vi "Load Config_Palette Data.vi"(7 "Target Folder":path, 8 "error in (no error)":errorcluster, 9 "Section (\"Default Palette Data\")":string="Default Palette Data", 10 "Palette Data in":T1={"Display Name Override"="", "View Format"=2, "Palette Width"=5, "Help Tag"="", "Help File Path"=path "", "Palette Description"=""} {"View Format" items=["Icons", "Text", "Icons and Text"]}, 11 "Refnum in":T3) -> (0 "error out":errorcluster, 2 "Palette Data out":T1={"Display Name Override"="", "View Format"=2, "Palette Width"=0, "Help Tag"="", "Help File Path"=path "", "Palette Description"=""} {"View Format" items=["Icons", "Text", "Icons and Text"]}, 3 "Refnum out":T3)   [LabVIEW 2019, in "AutoMenuCreator.lvlib"]
uses:
  AutoMenuCreator.lvlib
  Ctl/Ctl_Config_Palette Data.ctl
  <vilib>/Palette API/Palette Menu/Public Type Define/View Format.ctl
  <vilib>/Utility/config.llb/Config Data RefNum.ctl
  <vilib>/Utility/config.llb/NI_LVConfig.lvlib
  <vilib>/Utility/Data Type/NI_Data Type.lvlib
  <vilib>/Palette API/Palette Menu/Palette Menu.lvlib
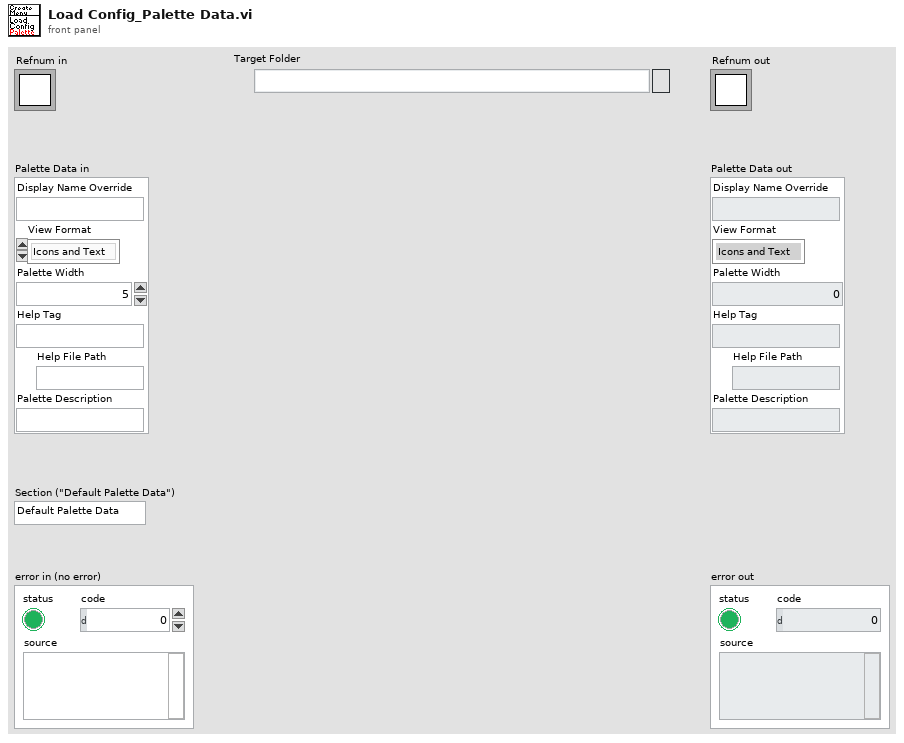
[diagram p1: front panel]
types:
  T1 = typedef "AutoMenuCreator.lvlib/Ctl_Config_Palette Data.ctl" = cluster{"Display Name Override":string, "View Format":T2, "Palette Width":i16, "Help Tag":string, "Help File Path":path, "Palette Description":string}
  T2 = typedef "Palette Menu.lvlib/View Format.ctl" = u16
  T3 = typedef "NI_LVConfig.lvlib/Config Data RefNum.ctl" = refnum<k1>
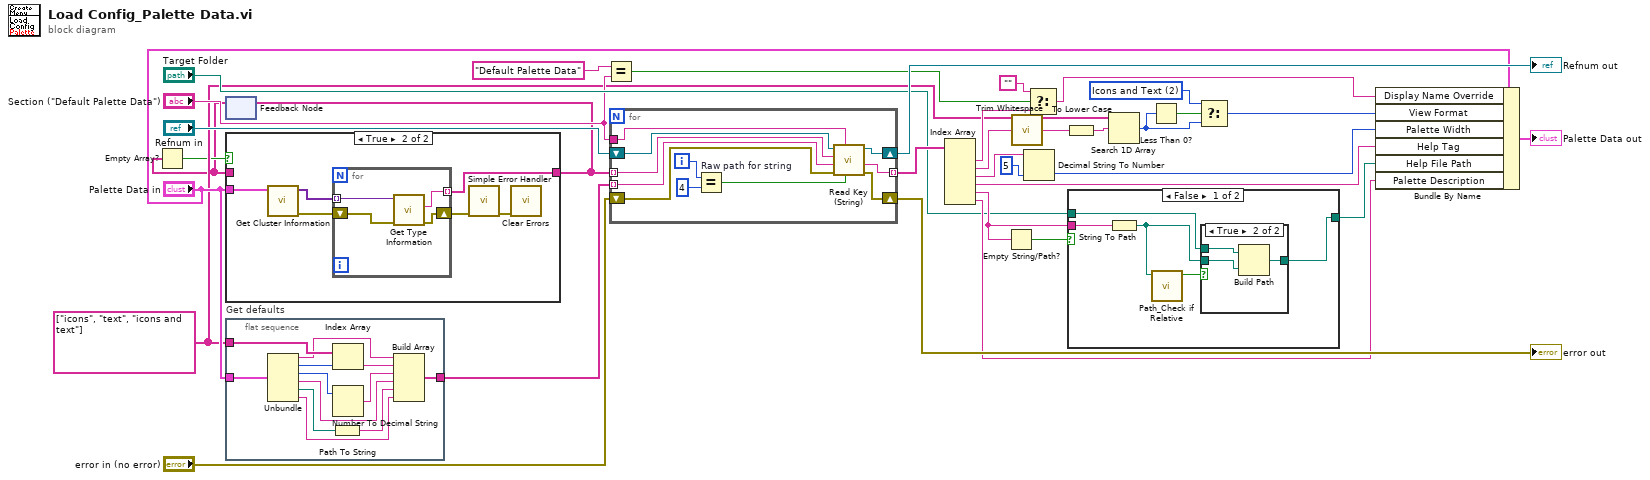
[diagram p0: block diagram]
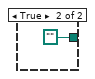
[diagram p4: hidden frame]
diagram:
  w6 = string[] ["icons", "text", "icons and text"]
  w20 = T2 2 items=["Icons", "Text", "Icons and Text"] ("View Format")
  n1 = feedback #1() -> (w1:string[])  [unwired: 1 in]
  n2 = Empty Array?(array=w1) -> (empty?=w2:bool)
  n3 = case shown="True" w2 {
    tunnel: "Palette Data in" -> [_ w41]
    tunnel: [w35 w38] -> w3
    tunnel: w1 -> [w35 _]
    frame False {
    }
    frame True {
      n4 = call <vilib>:"Get Cluster Information.vi"("variant"=w41) -> ("error out"=w39:errorcluster, "cluster elements"=w40:variant[])  [unwired: 9 in]
      n5 = for {
        tunnel: w40 -> [w45] mode=indexing
        tunnel: [w44] -> w38 mode=indexing
        shift-right: [w42] -> w37
        shift-left: w39 -> [w43]
        n6 = call <vilib>:"Get Type Information.vi"("error in (no error)"=w43, "variant"=w45) -> ("error out"=w42:errorcluster, "name"=w44:string)  [unwired: 5 in, 3 out]
      }
      n7 = call <vilib>:"Simple Error Handler.vi"("error in (no error)"=w37) -> ("error out"=w36:errorcluster)  [unwired: 4 in, 4 out]
      n8 = call <vilib>:"Clear Errors.vi"("error in (no error)"=w36) -> ()  [unwired: 5 in, 2 out]
    }
  }
  n9 = feedback-in #1(w3) -> ()
  n10 = flat-sequence "Get defaults" {
    tunnel: "Palette Data in" -> [w57]
    tunnel: w6 -> [w55]
    tunnel: [w46] -> w5
    frame #0 {
      n11 = Unbundle(w57) -> ("Display Name Override"=w54:string, "View Format"=w56:T2, "Palette Width"=w52:i16, "Help Tag"=w50:string, "Help File Path"=w49:path, "Palette Description"=w47:string)
      n12 = Path To String(path=w49) -> (string=w48:string)
      n13 = Index Array(array=w55, index=w56) -> (element=w53:string)
      n14 = Number To Decimal String(number=w52) -> (decimal integer string=w51:string)  [unwired: 1 in]
      n15 = Build Array(w54, w53, w51, w50, w48, w47) -> (w46:string[])
    }
  }
  n16 = Equal?(x="Default Palette Data" ("section"), y="Section (\"Default Palette Data\")") -> (x = y?=w11:bool)
  n17 = for {
    tunnel: "Section (\"Default Palette Data\")" -> [w67]
    tunnel: [w66] -> w30 mode=indexing
    shift-right: [w65] -> w32
    shift-left: "Refnum in" -> [w68]
    shift-right: [w64] -> w31
    shift-left: "error in (no error)" -> [w58]
    tunnel: w5 -> [w63] mode=indexing
    tunnel: w3 -> [w59] mode=indexing
    i -> [w62]
    n18 = Equal? "Raw path for string"(x=w62, y=4) -> (x = y?=w60:bool)
    n19 = call <vilib>:"Read Key (String).vi"("read raw string? (F)"=w60, "section"=w67, "error in (no error)"=w58, "default value"=w63, "key"=w59, "refnum"=w68) -> ("error out"=w64:errorcluster, "value"=w66:string, "refnum out"=w65:T3)  [unwired: 2 in, 1 out]
  }
  "error out" <- w31
  "Refnum out" <- w32
  n20 = Index Array(array=w30) -> (element #1=w9:string, element #2=w29:string, element #3=w27:string, element #4=w25:string, element #5=w17:string, element #6=w24:string)  [unwired: 6 in]
  n21 = Empty String/Path?(string/path=w17) -> (empty?=w16:bool)
  n22 = call <vilib>:"Trim Whitespace.vi"("string"=w29) -> ("trimmed string"=w23:string)  [unwired: 1 in]
  n23 = Decimal String To Number(string=w27, default (0L)=i16 5 ("default (0 I32)")) -> (number=w26:i16)  [unwired: 1 in, 1 out]
  n24 = Select(t="", s=w11, f=w9) -> (s? t:f=w8:string)
  n25 = To Lower Case(string=w23) -> (all lower case string=w22:string)
  n26 = case shown="False" w16 {
    tunnel: w17 -> [w71 _]
    tunnel: [w69 path ""] -> w15
    tunnel: "Target Folder" -> [w70 _]
    frame False {
      n27 = String To Path(string=w71) -> (path=w72:path)
      n28 = call "Path_Check if Relative.vi"("Path"=w72) -> ("Relative Path?"=w73:bool)  [unwired: 10 in]
      n29 = case shown="True" w73 {
        tunnel: w70 -> [_ w77]
        tunnel: w72 -> [w74 w76]
        tunnel: [w74 w75] -> w69
        frame False {
        }
        frame True {
          n30 = Build Path(base path=w77, name or relative path=w76) -> (appended path=w75:path)
        }
      }
    }
    frame True {
    }
  }
  n31 = Search 1D Array(1D array=w6, element=w22) -> (index of element=w19:i32)  [unwired: 1 in]
  n32 = Less Than 0?(x=w19) -> (x < 0?=w21:bool)
  n33 = Select(t=w20, s=w21, f=w19) -> (s? t:f=w18:i32)
  n34 = Bundle By Name(cluster="Palette Data in", "Display Name Override"=w8, "View Format"=w18, "Palette Width"=w26, "Help Tag"=w25, "Help File Path"=w15, "Palette Description"=w24) -> (→"Palette Data out":T1)
